vi "FROG_CenterPeak.vi"(1 "Input":dbl[][](array[numeric])) -> (0 "Output":dbl[][](array[numeric]))   [LabVIEW 2013]
panel:
  out "central pos":dbl
  out "max y pos":dbl
  out "max x pos":dbl
  out "y deviation":dbl
  out "x deviation":dbl
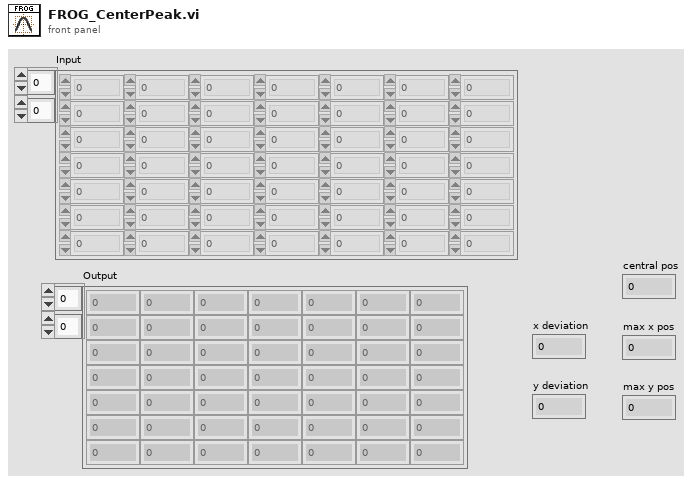
[diagram p1: front panel]
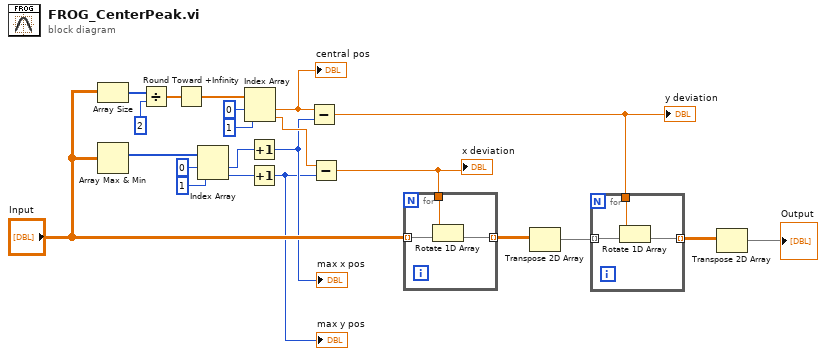
[diagram p0: block diagram]
diagram:
  n1 = Array Size(array="Input") -> (size(s)=w9:i32[])
  n2 = Array Max & Min(array="Input") -> (max index (indices)=w22:i32[])  [unwired: 3 out]
  n3 = Divide(x=w9, y=2) -> (x/y=w8:dbl[])
  n4 = Round Toward +Infinity(x=w8) -> (ceil(x): smallest int >= x=w1:dbl[])
  n5 = Index Array(array=w22, index #1=0 ("index"), index #2=1 ("index")) -> (element #1=w16:i32, element #2=w15:i32)
  n6 = Index Array(array=w1, index #1=0 ("index"), index #2=1 ("index")) -> (element #1=w4:dbl, element #2=w10:dbl)
  "central pos" <- w4
  n7 = Increment(x=w16) -> (x+1=w6:i32)
  "max x pos" <- w6
  n8 = Increment(x=w15) -> (x+1=w5:i32)
  "max y pos" <- w5
  n9 = Subtract(x=w4, y=w6) -> (x-y=w3:dbl)
  "y deviation" <- w3
  n10 = Subtract(x=w10, y=w5) -> (x-y=w2:dbl)
  "x deviation" <- w2
  n11 = for {
    tunnel: "Input" -> [w25] mode=indexing
    tunnel: w2 -> [w24]
    tunnel: [w23] -> w14 mode=indexing
    n12 = Rotate 1D Array(1:w25, 2:w24) -> (0:w23:dbl[])
  }
  n13 = Transpose 2D Array(2D array=w14) -> (transposed array=w12:dbl[][])
  n14 = for {
    tunnel: w12 -> [w28] mode=indexing
    tunnel: w3 -> [w27]
    tunnel: [w26] -> w13 mode=indexing
    n15 = Rotate 1D Array(1:w28, 2:w27) -> (0:w26:dbl[])
  }
  n16 = Transpose 2D Array(2D array=w13) -> (transposed array=→"Output":dbl[][])
